vi "FP_to_DSC.vi"(6 "Mode":u16, 7 "Configuration":T1={"FP port"="COM3", "MG port"="COM4", "PT Enabled?"=FALSE, "MG  channel P8"=65535, "Stop auto recovery if still is empty"=FALSE, "PT port"="COM2", "MG Enabled?"=FALSE, "Type"=enum."CF", "Slave Address"=16, "S1 Enabled?"=FALSE, "S1 port"="COM2", "S2 Enabled?"=FALSE, "S2 port"="COM2", "Device address S1"=1, "Device address S2"=2} {"MG  channel P8" items=["Channel 1", "Channel 2", "Channel 3", "Channel 4", "Channel 5", "Channel 6"]; "Slave Address" min=16 max=126 step=1}, 8 "FP Status Bits":u32[](array[numeric]), 9 "PT Data":dbl[](array[numeric]), 10 "MG Data":dbl[](array[numeric]), 11 "FP Data":sgl[](array[numeric])) -> ()   [LabVIEW 2013]
panel:
  # "MaxiGauge"
  # "Pulse Tube"
  # "Turbo 1 (S1) (Pfeiffer HiPACE only)"
  # "Turbo2 (S2) (Pfeiffer HiPACE only)"
  # "Front Panel"
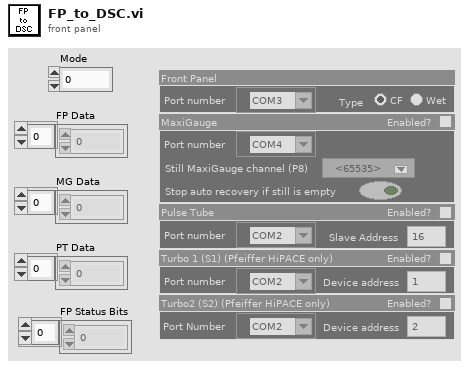
[diagram p1: front panel]
types:
  T1 = cluster{"FP port":refnum<visa-resource-name>, "MG port":refnum<visa-resource-name>, "PT Enabled?":bool, "MG  channel P8":u16, "Stop auto recovery if still is empty":bool, "PT port":refnum<visa-resource-name>, "MG Enabled?":bool, "Type":enum32{"CF", "Wet"}, "Slave Address":u8, "S1 Enabled?":bool, "S1 port":refnum<visa-resource-name>, "S2 Enabled?":bool, "S2 port":refnum<visa-resource-name>, "Device address S1":u8, "Device address S2":u8}
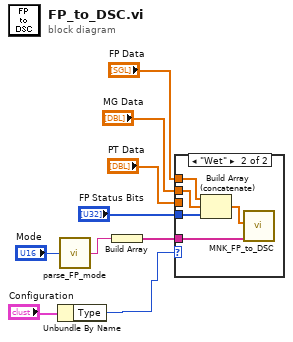
[diagram p0: block diagram]
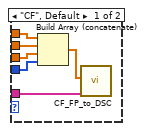
[diagram p2: hidden frame]
diagram:
  n1 = Unbundle By Name("Configuration") -> ("Type"=w1:enum32{"CF", "Wet"})
  n2 = call "parse_FP_mode.vi"("line index"="Mode") -> ("output string"=w8:string)
  n3 = Build Array(w8) -> (w9:string[])
  n4 = case shown="\"Wet\"" w1 {
    tunnel: "FP Data" -> [w14 w20]
    tunnel: "MG Data" -> [w13 w19]
    tunnel: "PT Data" -> [w12 _]
    tunnel: w9 -> [w11 w16]
    tunnel: "FP Status Bits" -> [w10 w18]
    frame "CF", Default {
      n5 = Build Array (concatenate)(w14, w13, w12, w10) -> (w15:dbl[])
      n6 = call "CF_FP_to_DSC.vi"("str"=w11, "dbl"=w15) -> ()  [unwired: 2 in]
    }
    frame "Wet" {
      n7 = Build Array (concatenate)(w20, w19, w18) -> (w17:dbl[])
      n8 = call "MNK_FP_to_DSC.vi"("str"=w16, "dbl"=w17) -> ()  [unwired: 2 in]
    }
  }
